vi "Read Control to write_.vi"(8 "error in (no error)":errorcluster, 11 "Modbus in":refnum<class "Modbus.lvclass">) -> (0 "error out":errorcluster, 2 "Control to write?":bool, 3 "Modbus out":refnum<class "Modbus.lvclass">)   [LabVIEW 2020, in "Modbus.lvlib" / "Modbus.lvclass"]
uses:
  Modbus.lvclass
  Modbus.lvclass/Modbus.ctl
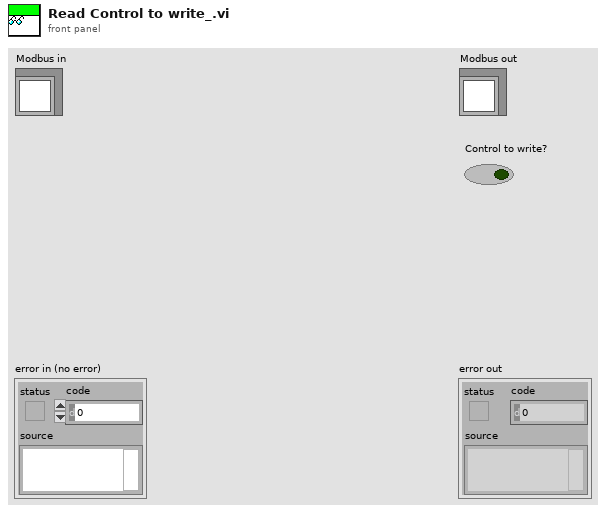
[diagram p1: front panel]
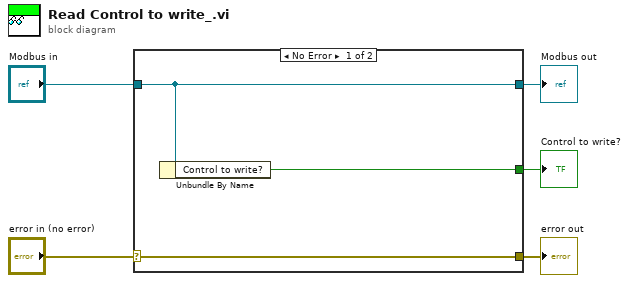
[diagram p0: block diagram]
diagram:
  n1 = case shown="No Error" "error in (no error)" {
    selector: "error in (no error)" -> [w8 w9]
    tunnel: [w8 w9] -> w4
    tunnel: [w7 w10] -> w2
    tunnel: "Modbus in" -> [w7 w10]
    tunnel: [w6 _] -> w1
    frame No Error {
      n2 = Unbundle By Name(w7) -> ("Control to write?"=w6:bool)
    }
    frame Error {
    }
  }
  "error out" <- w4
  "Modbus out" <- w2
  "Control to write?" <- w1
